vi "get_mean_speed_from_gpx_speed.vi"(9 "to":dbl format="%#_13g", 10 "from":dbl format="%#_13g", 11 "speed":cluster{timestamp[], dbl[]}(graph)) -> (0 "true dt":dbl format="%0.2f", 1 "true end time":dbl format="%0.2f", 2 "true start time":dbl format="%0.2f", 3 "mean":dbl format="%0.2f")   [LabVIEW 2020]
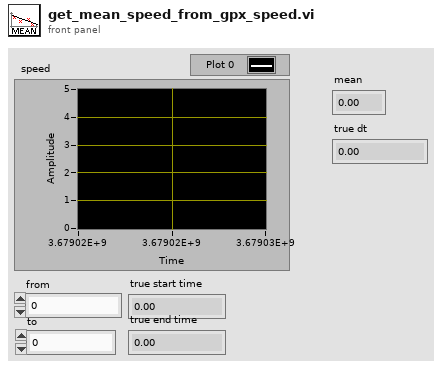
[diagram p1: front panel]
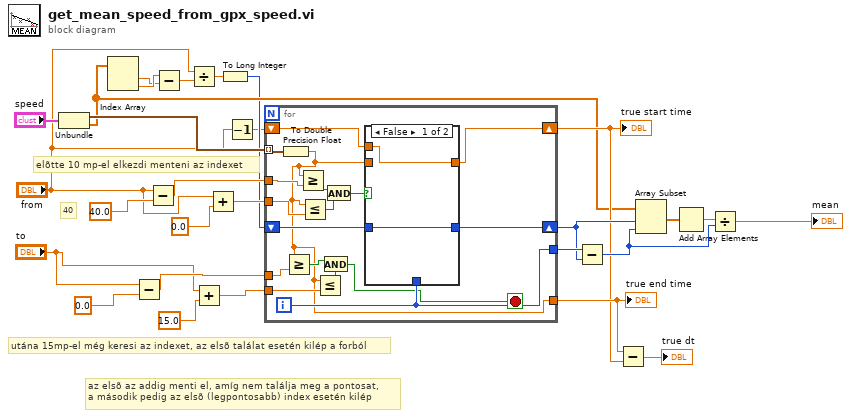
[diagram p0: block diagram]
diagram:
  # "40"
  # "az elsõ az addig menti el, amíg nem találja meg a pontosat,\na második pedig az elsõ (legpontosabb) index esetén kilép"
  # "utána 15mp-el még keresi az indexet, az elsõ találat esetén kilép a forból"
  # "elõtte 10 mp-el elkezdi menteni az indexet"
  n1 = Unbundle("speed") -> (w27:timestamp[], w8:dbl[])
  n2 = Index Array(array=w8) -> (element #1=w6:dbl, element #2=w7:dbl)  [unwired: 2 in]
  n3 = Subtract(x="to", y=0.0) -> (x-y=w14:dbl)
  n4 = Subtract(x="from", y=40.0) -> (x-y=w17:dbl)
  n5 = Subtract(x=w7, y=w6) -> (x-y=w5:dbl)
  n6 = Divide(x="from", y=w5) -> (x/y=w4:dbl)
  n7 = Add(x="to", y=15.0) -> (x+y=w13:dbl)
  n8 = Add(x="from", y=0.0) -> (x+y=w19:dbl)
  n9 = To Long Integer(number=w4) -> (32bit integer=w3:i32)
  n10 = Decrement(x="from") -> (x-1=w2:dbl)
  n11 = for {
    tunnel: w17 -> [w38]
    tunnel: w27 -> [w45] mode=indexing
    shift-right: [w44] -> w25
    shift-left: w3 -> [w43]
    tunnel: w14 -> [w37]
    tunnel: [w42] -> w26
    tunnel: w19 -> [w33]
    tunnel: w13 -> [w32]
    shift-right: [w31] -> w10
    shift-left: w2 -> [w29]
    tunnel: [w30] -> w11
    i -> [w42]
    stop <- w34 stop-if-true
    n12 = To Double Precision Float(number=w45) -> (double precision float=w30:dbl)
    n13 = Greater Or Equal?(x=w30, y=w37) -> (x >= y?=w36:bool)
    n14 = Greater Or Equal?(x=w30, y=w38) -> (x >= y?=w40:bool)
    n15 = Less Or Equal?(x=w30, y=w33) -> (x <= y?=w39:bool)
    n16 = Less Or Equal?(x=w30, y=w32) -> (x <= y?=w35:bool)
    n17 = And(x=w36, y=w35) -> (x .and. y?=w34:bool)
    n18 = And(x=w40, y=w39) -> (x .and. y?=w41:bool)
    n19 = case shown="False" w41 {
      tunnel: [w47 w49] -> w44
      tunnel: w42 -> [_ w49]
      tunnel: w43 -> [w47 _]
      tunnel: w30 -> [_ w48]
      tunnel: [w46 w48] -> w31
      tunnel: w29 -> [w46 _]
      frame False {
      }
      frame True {
      }
    }
  }
  "true start time" <- w10
  "true end time" <- w11
  n20 = Subtract(x=w26, y=w25) -> (x-y=w21:i32)
  n21 = Subtract(x=w11, y=w10) -> (x-y=→"true dt":dbl)
  n22 = Array Subset(array=w8, index=w25, length=w21) -> (w24:dbl[])
  n23 = Add Array Elements(numeric array=w24) -> (sum=w23:dbl)
  n24 = Divide(x=w23, y=w21) -> (x/y=→"mean":dbl)
